vi "Ballard - 1553 Asynchronous RT Driver VI.vi"(10 "Parameters":variant, 11 "Process":refnum<class "Process.lvclass">) -> ()   [LabVIEW 2020, in "Ballard MIL-1553 Engine.lvlib"]
doc: "This VI is the Asynchronous VI for RT part."
uses:
  Ballard MIL-1553 Engine.lvlib
  <vilib>/NI/NIVS Inline Async API/_VS Inline Async API/Process/Process.lvclass
  <vilib>/NI/NIVS Inline Async API/_VS Inline Async API/Process/Process.lvclass/Process.ctl
  Controls/RT Async Data.ctl
  Controls/RT Async_Map BC2RT.ctl
  <vilib>/NI VeriStand/Custom Device API/Data Reference.ctl
  Controls/RT Async_Map_Type.ctl
  Controls/RT Async_Raw Values.ctl
  Controls/RT Async_Raw Values to Messages Index_Association.ctl
  Controls/Asynchronous - Parameter map_type.ctl
  Shared/EncodeDecode/_typedefs/parameter_config_type.ctl
  Shared/EncodeDecode/_typedefs/parameter_config_type_type.ctl
  Shared/EncodeDecode/_typedefs/parameter_config_encoding_type.ctl
  Controls/RT Async_Map RT2BC.ctl
  Controls/RT Async_Map RTs Status.ctl
  Controls/RT Async_Map BC Command Channels.ctl
  <vilib>/NI VeriStand/Custom Device API/Custom Device Item Ref.ctl
  Controls/RT Async_Map BC Acyclic Messages Trigger.ctl
  Controls/RT Async_Map RT Command Channels.ctl
  <vilib>/NI/NIVS Inline Async API/_Data Access Engine/Access Type Classes/Read/Read.lvclass/Read.ctl
  <vilib>/NI/NIVS Inline Async API/_Data Access Engine/Access Type Classes/ReadWrite/ReadWrite.lvclass/ReadWrite.ctl
  <vilib>/NI/NIVS Inline Async API/_Data Access Engine/Access Type Classes/Write/Write.lvclass/Write.ctl
  <vilib>/NI/NIVS Inline Async API/_Data Access Engine/Data Access Engine/Methods/Read.Data.Detect.vi
  <vilib>/NI/NIVS Inline Async API/_Data Access Engine/Data Access Engine/Methods/ReadWrite.Data.Read.vi
  <vilib>/NI/NIVS Inline Async API/_Data Access Engine/Data Access Engine/Methods/ReadWrite.Data.Reset.vi
  <vilib>/NI/NIVS Inline Async API/_Data Access Engine/Data Access Engine/Methods/Write.Data.vi
  <vilib>/NI/NIVS Inline Async API/_Data Access Engine/Data Access Engine/Methods/Read.Data.vi
  <vilib>/NI/NIVS Inline Async API/_VS Inline Async API/Process/Data Member Access/Read Data Access.vi
  <vilib>/NI/NIVS Inline Async API/_VS Inline Async API/Error Handling Process/SubVIs/Error.ConvertArray.vi
  <vilib>/NI/NIVS Inline Async API/_Data Access Engine/Access Type Classes/Read/Read.ProcessData.Detect.vi
  <vilib>/NI/NIVS Inline Async API/_Data Access Engine/Access Type Classes/ReadWrite/ReadWrite.ProcessData.Read.vi
  <vilib>/NI/NIVS Inline Async API/_Data Access Engine/Access Type Classes/ReadWrite/ReadWrite.ProcessData.Reset.vi
  <vilib>/NI/NIVS Inline Async API/_Data Access Engine/Access Type Classes/Write/Write.ProcessData.vi
  <vilib>/NI/NIVS Inline Async API/_Data Access Engine/Access Type Classes/Read/Read.ProcessData.vi
  <vilib>/NI/NIVS Inline Async API/_Data Access Engine/Access Type Classes/Write/Write.Buffer.vi
  <vilib>/NI/NIVS Inline Async API/_Data Access Engine/Access Type Classes/Write/Write.Commit.vi
  <vilib>/NI/NIVS Inline Async API/_Data Access Engine/Data Access Engine/Methods/Read.Lookup.vi
  <vilib>/NI/NIVS Inline Async API/_Data Access Engine/Data Access Engine/Methods/ReadWrite.Lookup.vi
  <vilib>/NI/NIVS Inline Async API/_Data Access Engine/Data Access Engine/Methods/Write.Lookup.vi
  <vilib>/NI/NIVS Inline Async API/_Data Access Engine/Data Access Engine/Data Access Engine.lvclass
  <vilib>/NI VeriStand/Custom Device API/Custom Device API.lvlib
panel:
  # "Custom Device Template\nv1.0"
  # "Use this template as a starting point for creating a custom device code module. The input controls shown here are specially named controls that the system will use to provide the device loop with data. The controls are not required for the device loop to run. For instance, if the device doesn't produce any output data, then you don't need the Device Outputs FIFO control. If you do use these controls, however, they need to have these exact names to be functional."
  # "The optional status notifier element is used to notify the RT engine of the last state of the custom device, and to indicate the device has completed execution. If this control is not used, a default No Error value is returned to the system when the device finishes execution.\n\nNote: This error state is not checked until the system shuts down. Use an output status channel to send more immediate status values to the system."
  # "This optional input can be used to send the VeriStand Engine the final status of the custom device initalization process. If this control exists on the custom device front panel, the VeriStand Engine will wait for a status update before starting up. If the custom device reports an error, that will abort the execution of the current configuration in the VeriStand Engine.\n\nThis control can be deleted if the custom device does not need to send the initialization status update."
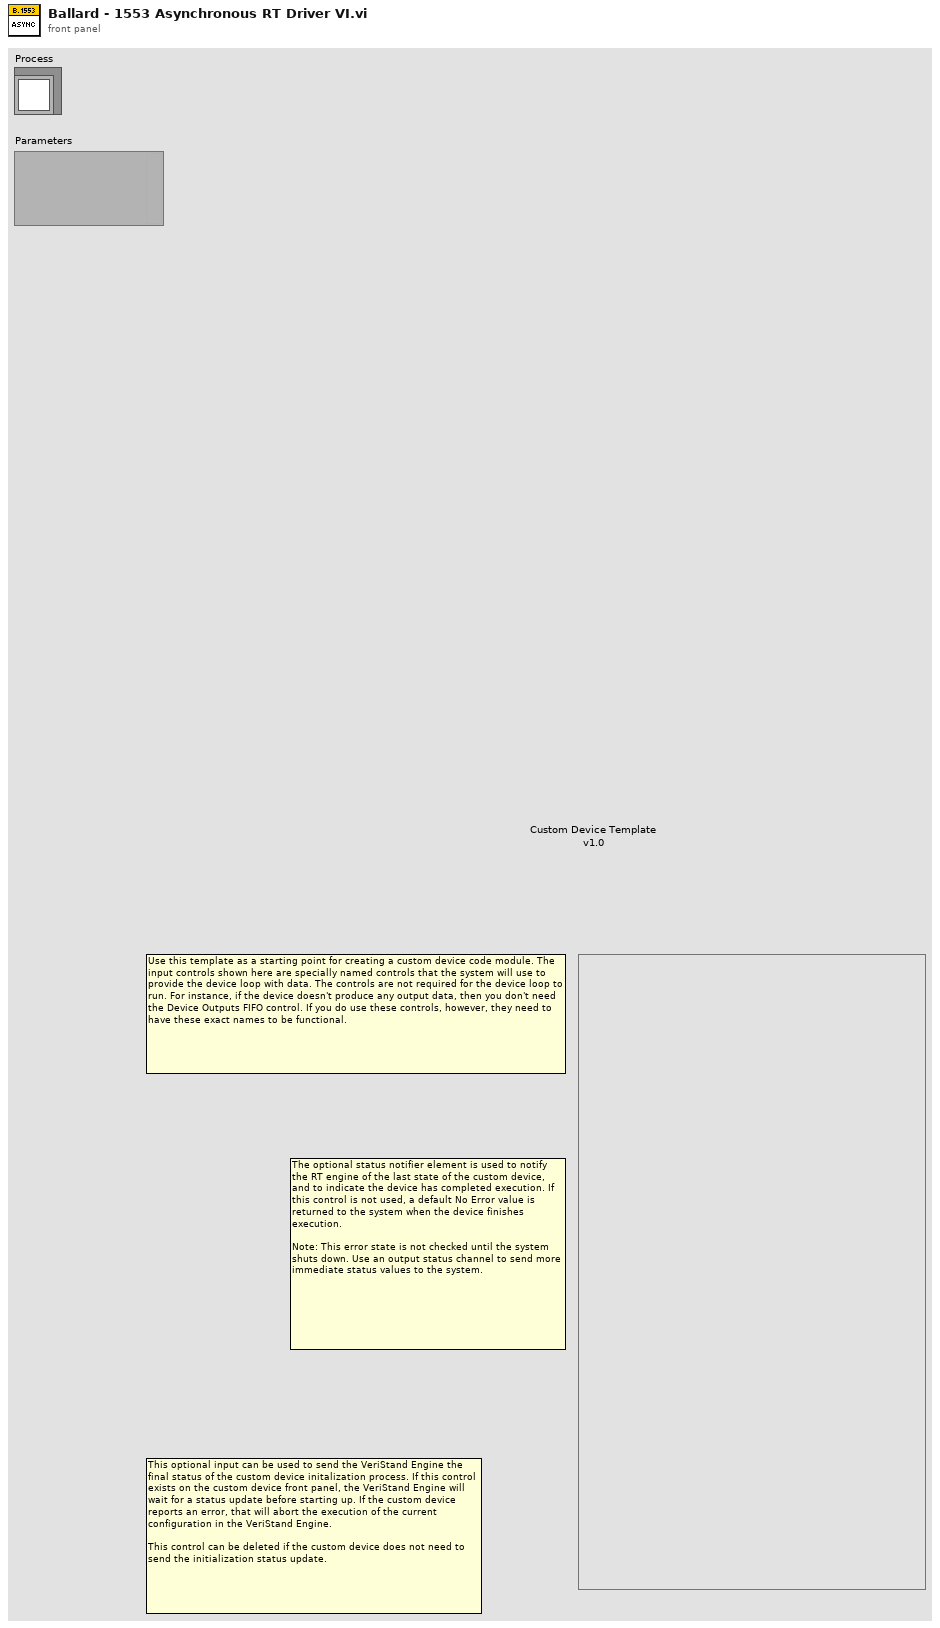
[diagram p1: front panel]
types:
  T1 = typedef "Ballard MIL-1553 Engine.lvlib/RT Async Data.ctl" = cluster{"Map (BC to RT)":T2[], "Raw Values (BC to RT)":T5, "param map (BC to RT)":T7, "Map (RT to ..)":T11[], "Raw Values (RT to ..)":T5, "param map (RT to BC)":T7, "Map (RTs Status)":T12[], "Raw Values (RTs Status)":T5, "Map (Bc Command Channels)":T13[], "MAP (BC Acyclic Messages Trigger)":T15[], "Map (RT Command Channels)":T16[], "Map (MC Rx)":T2[], "Raw Values (MC Rx)":T5, "param map (MC Rx)":T7, "Raw Values (MC Tx)":T5, "Map (MC Tx)":T11[], "param map (MC Tx)":T7}
  T2 = typedef "Ballard MIL-1553 Engine.lvlib/RT Async_Map BC2RT.ctl" = cluster{"Channel Index":i32, "ID":i32, "Channel Data Reference":T3, "Word Index":i32, "Message Handle":u64, "Type":T4, "Word Count":i32, "First Element Index":i32}
  T3 = typedef "Custom Device API.lvlib/Data Reference.ctl" = i32
  T4 = typedef "Ballard MIL-1553 Engine.lvlib/RT Async_Map_Type.ctl" = enum16{"Word (BC to RT)", "Word (MC (Rx))", "Acyclic Message Trigger", "Word (RT to ..)", "Word (RT to RT)", "Word (MC (Tx))", "RT Status", "BC Commands", "RT Commands"}
  T5 = typedef "Ballard MIL-1553 Engine.lvlib/RT Async_Raw Values.ctl" = cluster{"Association":T6[], "Raw Values Array":u16[]}
  T6 = typedef "Ballard MIL-1553 Engine.lvlib/RT Async_Raw Values to Messages Index_Association.ctl" = cluster{"Message Index":i32, "Raw Value Index":i32}
  T7 = typedef "Ballard MIL-1553 Engine.lvlib/Asynchronous - Parameter map_type.ctl" = cluster{"ParamConfig":T8[], "word_count":u8[]}
  T8 = typedef "parameter_config_type.ctl" = cluster{"Name":string, "Type":T9, "Units":string, "Nword":i32, "StartBit":i32, "Size":i32, "LSB_Value":i32, "Offset":i32, "Encoding":T10}
  T9 = typedef "parameter_config_type_type.ctl" = enum16{"Opaque", "Enum", "Float", "Integer", "Bcd", "Bool"}
  T10 = typedef "parameter_config_encoding_type.ctl" = enum16{"None", "2-complement", "Unsigned"}
  T11 = typedef "Ballard MIL-1553 Engine.lvlib/RT Async_Map RT2BC.ctl" = cluster{"Channel Index":i32, "ID":i32, "Word Data Reference":T3, "First element Index":i32, "rt Transfer Handle":u64, "Type":T4, "Word Count":i32}
  T12 = typedef "Ballard MIL-1553 Engine.lvlib/RT Async_Map RTs Status.ctl" = cluster{"Channel Index":i32, "ID":i32, "rt Transfer Handle":u64, "Type":T4}
  T13 = typedef "Ballard MIL-1553 Engine.lvlib/RT Async_Map BC Command Channels.ctl" = cluster{"Channel Index":i32, "ID":i32, "BC Handle":u64, "Type":T4, "BC Command Channel Ref":T14, "Command Type":enum16{"Start Command", "Stop Command"}}
  T14 = typedef "Custom Device API.lvlib/Custom Device Item Ref.ctl" = u64
  T15 = typedef "Ballard MIL-1553 Engine.lvlib/RT Async_Map BC Acyclic Messages Trigger.ctl" = cluster{"Channel Index":i32, "BC Handle":u64, "Type":T4, "Acyclic Message Trigger Channel Ref":T14, "Message Name":string}
  T16 = typedef "Ballard MIL-1553 Engine.lvlib/RT Async_Map RT Command Channels.ctl" = cluster{"Channel Index":i32, "ID":i32, "RT Handle":u64, "Type":T4, "RT Command Channel Ref":T14, "Command Type":enum16{"Start Command", "Stop Command"}}
  T17 = typedef "Data Access Engine.lvlib/Data Access Engine.lvclass/Read.DVR.ctl" = refnum<data-value>
  T18 = typedef "Data Access Engine.lvlib/Data Access Engine.lvclass/ReadWrite.DVR.ctl" = refnum<data-value>
  T19 = typedef "Data Access Engine.lvlib/Data Access Engine.lvclass/Write.DVR.ctl" = refnum<data-value>
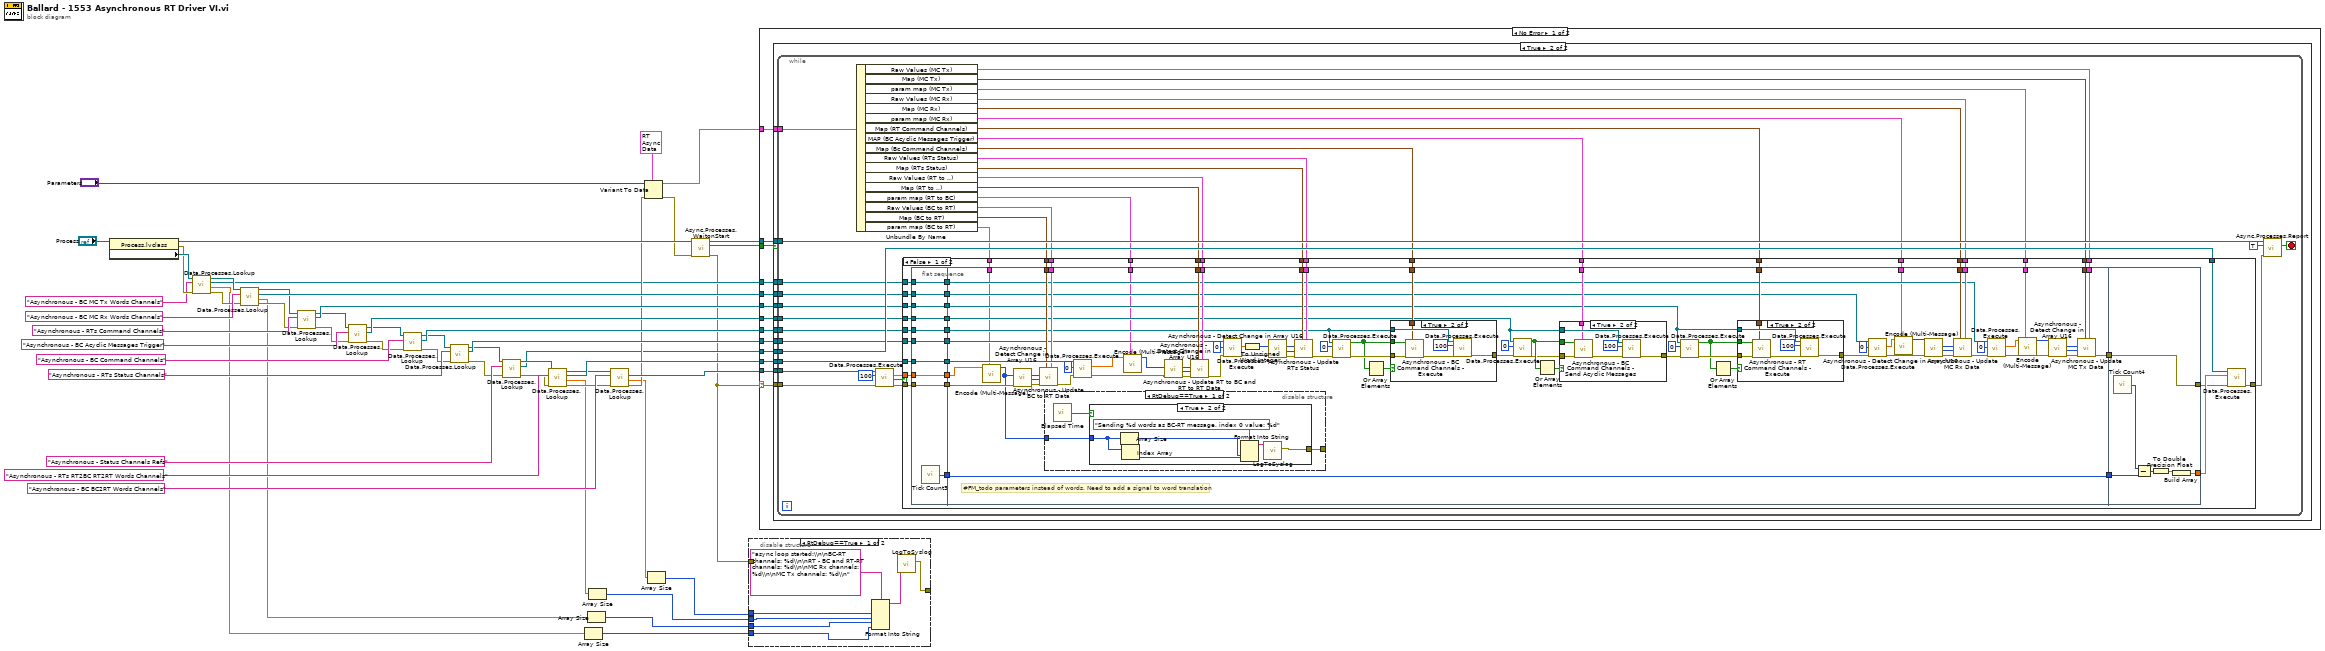
[diagram p0: block diagram]
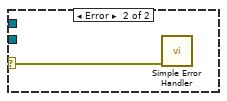
[diagram p10: hidden frame]
diagram:
  n1 = property class="Process.lvclass"(reference="Process") -> (reference out=w50:refnum<class "Process.lvclass">, error out=w15:errorcluster, "Data Member Access:Data Access"=w16:refnum<class "Data Access Engine.lvclass">)  [unwired: 1 in]
  n2 = call-poly <vilib>:"Data.Processes.Lookup.vi"("error in (no error)"=w15, "Name"="Asynchronous - BC MC Tx Words Channels", "Data Access API in"=w16) -> ("error out"=w14:errorcluster, "Initial Values"=w8:dbl[], "Ref"=w12:T17, "Data Access API out"=w13:refnum<class "Data Access Engine.lvclass">)  [unwired: 5 in]
  n3 = call-poly <vilib>:"Data.Processes.Lookup.vi"("error in (no error)"=w14, "Name"="Asynchronous - BC MC Rx Words Channels", "Data Access API in"=w13) -> ("error out"=w17:errorcluster, "Initial Values"=w7:dbl[], "Ref"=w32:T17, "Data Access API out"=w18:refnum<class "Data Access Engine.lvclass">)  [unwired: 5 in]
  n4 = call-poly <vilib>:"Data.Processes.Lookup.vi"("error in (no error)"=w17, "Name"="Asynchronous - RTs Command Channels", "Data Access API in"=w18) -> ("error out"=w19:errorcluster, "Ref"=w34:T18, "Data Access API out"=w20:refnum<class "Data Access Engine.lvclass">)  [unwired: 5 in, 1 out]
  n5 = call-poly <vilib>:"Data.Processes.Lookup.vi"("error in (no error)"=w19, "Name"="Asynchronous - BC Acyclic Messages Trigger", "Data Access API in"=w20) -> ("error out"=w22:errorcluster, "Ref"=w36:T18, "Data Access API out"=w21:refnum<class "Data Access Engine.lvclass">)  [unwired: 5 in, 1 out]
  n6 = call-poly <vilib>:"Data.Processes.Lookup.vi"("error in (no error)"=w22, "Name"="Asynchronous - BC Command Channels", "Data Access API in"=w21) -> ("error out"=w23:errorcluster, "Ref"=w38:T18, "Data Access API out"=w24:refnum<class "Data Access Engine.lvclass">)  [unwired: 5 in, 1 out]
  n7 = call-poly <vilib>:"Data.Processes.Lookup.vi"("error in (no error)"=w23, "Name"="Asynchronous - RTs Status Channels", "Data Access API in"=w24) -> ("error out"=w25:errorcluster, "Ref"=w40:T17, "Data Access API out"=w26:refnum<class "Data Access Engine.lvclass">)  [unwired: 5 in, 1 out]
  n8 = call-poly <vilib>:"Data.Processes.Lookup.vi"("error in (no error)"=w25, "Name"="Asynchronous - Status Channels Refs", "Data Access API in"=w26) -> ("error out"=w27:errorcluster, "Ref"=w10:T19, "Data Access API out"=w28:refnum<class "Data Access Engine.lvclass">)  [unwired: 5 in, 1 out]
  n9 = call-poly <vilib>:"Data.Processes.Lookup.vi"("error in (no error)"=w27, "Name"="Asynchronous - RTs RT2BC RT2RT Words Channels", "Data Access API in"=w28) -> ("error out"=w29:errorcluster, "Initial Values"=w6:dbl[], "Ref"=w46:T17, "Data Access API out"=w44:refnum<class "Data Access Engine.lvclass">)  [unwired: 5 in]
  n10 = Array Size(array=w8) -> (size(s)=w1:i32)
  n11 = Array Size(array=w7) -> (size(s)=w2:i32)
  n12 = Array Size(array=w6) -> (size(s)=w3:i32)
  n13 = call-poly <vilib>:"Data.Processes.Lookup.vi"("error in (no error)"=w29, "Name"="Asynchronous - BC BC2RT Words Channels", "Data Access API in"=w44) -> ("error out"=w30:errorcluster, "Initial Values"=w5:dbl[], "Ref"=w52:T17)  [unwired: 5 in, 1 out]
  n14 = Variant To Data(error in=w30, type=T1 {"Map (BC to RT)"=[], "Raw Values (BC to RT)"={"Association"=[], "Raw Values Array"=[]}, "param map (BC to RT)"={"ParamConfig"=[], "word_count"=[]}, "Map (RT to ..)"=[], "Raw Values (RT to ..)"={"Association"=[], "Raw Values Array"=[]}, "param map (RT to BC)"={"ParamConfig"=[], "word_count"=[]}, "Map (RTs Status)"=[], "Raw Values (RTs Status)"={"Association"=[], "Raw Values Array"=[]}, "Map (Bc Command Channels)"=[], "MAP (BC Acyclic Messages Trigger)"=[], "Map (RT Command Channels)"=[], "Map (MC Rx)"=[], "Raw Values (MC Rx)"={"Association"=[], "Raw Values Array"=[]}, "param map (MC Rx)"={"ParamConfig"=[], "word_count"=[]}, "Raw Values (MC Tx)"={"Association"=[], "Raw Values Array"=[]}, "Map (MC Tx)"=[], "param map (MC Tx)"={"ParamConfig"=[], "word_count"=[]}} ("RT Async Data"), Variant="Parameters") -> (data=w45:T1, error out=w31:errorcluster)
  n15 = Array Size(array=w5) -> (size(s)=w4:i32)
  n16 = call <vilib>:"Async.Processes.WaitonStart.vi"("error in (no error)"=w31, "Process"=w50) -> ("error out"=w9:errorcluster, "Execute"=w54:bool, "Process out"=w53:refnum<class "Process.lvclass">)  [unwired: 7 in]
  n17 = disable-structure shown="RtDebug==True" {
    disable-tunnel: [w59 _] -> _
    disable-tunnel: w9 -> [_ _]
    disable-tunnel: w4 -> [w58 _]
    disable-tunnel: w3 -> [w57 _]
    disable-tunnel: w2 -> [w56 _]
    disable-tunnel: w1 -> [w55 _]
    frame condition #0 (active) {
      n18 = Format Into String(format string="async loop started:\\n\nBC-RT channels: %d\\n\nRT - BC and RT-RT channels: %d\\n\nMC Rx channels: %d\\n\nMC Tx channels: %d\\n", w58, w57, w56, w55) -> (resulting string=w61:string)  [unwired: 2 in, 1 out]
      n19 = call "LogToSyslog.vi"("message"=w61) -> ("error out"=w59:errorcluster)  [unwired: 9 in, 1 out]
    }
    frame condition #1 {
    }
  }
  n20 = case shown="No Error" w9 {
    selector: w9 -> [w70 w294]
    tunnel: w54 -> [w74 _]
    tunnel: w53 -> [w73 _]
    tunnel: w10 -> [w72 _]
    tunnel: w52 -> [w71 _]
    tunnel: w45 -> [w69 _]
    tunnel: w46 -> [w68 _]
    tunnel: w40 -> [w67 _]
    tunnel: w38 -> [w66 _]
    tunnel: w36 -> [w65 _]
    tunnel: w34 -> [w64 _]
    tunnel: w32 -> [w63 _]
    tunnel: w12 -> [w62 _]
    frame No Error {
      n21 = case shown="True" w74 {
        tunnel: w70 -> [_ w83]
        tunnel: w73 -> [_ w84]
        tunnel: w71 -> [_ w86]
        tunnel: w72 -> [_ w85]
        tunnel: w69 -> [_ w82]
        tunnel: w68 -> [_ w81]
        tunnel: w67 -> [_ w80]
        tunnel: w66 -> [_ w79]
        tunnel: w65 -> [_ w78]
        tunnel: w64 -> [_ w77]
        tunnel: w63 -> [_ w76]
        tunnel: w62 -> [_ w75]
        frame False {
        }
        frame True {
          n22 = while {
            tunnel: w83 -> [w118]
            tunnel: w84 -> [w122]
            tunnel: w86 -> [w120]
            tunnel: w85 -> [w119]
            tunnel: w82 -> [w115]
            tunnel: w81 -> [w114]
            tunnel: w80 -> [w107]
            tunnel: w79 -> [w104]
            tunnel: w78 -> [w102]
            tunnel: w77 -> [w100]
            tunnel: w76 -> [w98]
            tunnel: w75 -> [w93]
            stop <- w121 stop-if-true
            n23 = Unbundle By Name(w115) -> ("Raw Values (MC Tx)"=w91:T5, "Map (MC Tx)"=w92:T11[], "param map (MC Tx)"=w87:T7, "Raw Values (MC Rx)"=w95:T5, "Map (MC Rx)"=w94:T2[], "param map (MC Rx)"=w88:T7, "Map (RT Command Channels)"=w99:T16[], "MAP (BC Acyclic Messages Trigger)"=w101:T15[], "Map (Bc Command Channels)"=w103:T13[], "Raw Values (RTs Status)"=w105:T5, "Map (RTs Status)"=w106:T12[], "Raw Values (RT to ..)"=w110:T5, "Map (RT to ..)"=w111:T11[], "param map (RT to BC)"=w89:T7, "Raw Values (BC to RT)"=w108:T5, "Map (BC to RT)"=w109:T2[], "param map (BC to RT)"=w90:T7)
            n24 = call-poly <vilib>:"Data.Processes.Execute.vi"("error in (no error)"=w118, "timeout ms"=100, "Ref"=w120) -> ("error out"=w116:errorcluster, "Timeout?"=w113:bool, "Values"=w117:dbl[])  [unwired: 6 in]
            n25 = case shown="False" w113 {
              tunnel: w119 -> [w159 _]
              tunnel: [w158 w293] -> w97
              tunnel: w117 -> [w157 _]
              tunnel: w116 -> [w156 w293]
              tunnel: w114 -> [w154 _]
              tunnel: w111 -> [w153 _]
              tunnel: w110 -> [w152 _]
              tunnel: w109 -> [w151 _]
              tunnel: w108 -> [w150 _]
              tunnel: w107 -> [w149 _]
              tunnel: w106 -> [w147 _]
              tunnel: w105 -> [w146 _]
              tunnel: w104 -> [w145 _]
              tunnel: w103 -> [w142 _]
              tunnel: w102 -> [w141 _]
              tunnel: w101 -> [w139 _]
              tunnel: w100 -> [w138 _]
              tunnel: w99 -> [w136 _]
              tunnel: w98 -> [w135 _]
              tunnel: w95 -> [w132 _]
              tunnel: w94 -> [w131 _]
              tunnel: w93 -> [w130 _]
              tunnel: w92 -> [w128 _]
              tunnel: w91 -> [w127 _]
              tunnel: w90 -> [w126 _]
              tunnel: w89 -> [w125 _]
              tunnel: w88 -> [w124 _]
              tunnel: w87 -> [w123 _]
              frame False {
                n26 = flat-sequence {
                  tunnel: w157 -> [w173]
                  tunnel: w156 -> [w174]
                  tunnel: [w174] -> w164
                  tunnel: [w173] -> w163
                  tunnel: [w172] -> w162
                  tunnel: w154 -> [w171]
                  tunnel: [w171] -> w161
                  tunnel: w149 -> [w170]
                  tunnel: [w170] -> w148
                  tunnel: w145 -> [w169]
                  tunnel: [w169] -> w144
                  tunnel: w141 -> [w168]
                  tunnel: [w168] -> w140
                  tunnel: w138 -> [w167]
                  tunnel: [w167] -> w137
                  tunnel: w135 -> [w166]
                  tunnel: [w166] -> w134
                  tunnel: w130 -> [w165]
                  tunnel: [w165] -> w129
                  tunnel: w164 -> [w249]
                  tunnel: w163 -> [w184]
                  tunnel: w162 -> [w253]
                  tunnel: [w253] -> w160
                  tunnel: w161 -> [w252]
                  tunnel: w153 -> [w251]
                  tunnel: w152 -> [w250]
                  tunnel: w151 -> [w245]
                  tunnel: w150 -> [w244]
                  tunnel: w148 -> [w242]
                  tunnel: w147 -> [w241]
                  tunnel: w146 -> [w240]
                  tunnel: w144 -> [w239]
                  tunnel: w142 -> [w238]
                  tunnel: w140 -> [w237]
                  tunnel: w139 -> [w236]
                  tunnel: w137 -> [w235]
                  tunnel: w136 -> [w234]
                  tunnel: w134 -> [w233]
                  tunnel: [w188] -> w133
                  tunnel: w132 -> [w197]
                  tunnel: w131 -> [w196]
                  tunnel: w129 -> [w187]
                  tunnel: w128 -> [w186]
                  tunnel: w127 -> [w185]
                  tunnel: w126 -> [w183]
                  tunnel: w125 -> [w180]
                  tunnel: w124 -> [w178]
                  tunnel: w123 -> [w176]
                  tunnel: w160 -> [w292]
                  tunnel: [w288] -> w155
                  tunnel: [w287] -> w143
                  tunnel: w133 -> [w287]
                  frame #0 {
                    n27 = call "Tick Count3"() -> ("Tick Count(uSec)"=w172:u32)
                  }
                  frame #1 {
                    # "#FM_todo parameters instead of words. Need to add a signal to word translation"
                    n28 = call "Encode (Multi-Message).vi"("param map"=w183, "parameters in"=w184) -> ("words out"=w175:u16[])  [unwired: 9 in]
                    n29 = call "Asynchronous - Detect Change in Array U16.vi"("Error (in)"=w249, "Data (in)"=w175) -> ("Error (out)"=w248:errorcluster, "Indexes"=w246:i32[], "Data (out)"=w247:u16[])  [unwired: 7 in]
                    n30 = call "Asynchronous - Update BC to RT Data.vi"("Raw Values (BC to RT)"=w244, "Map (BC to RT)"=w245, "Error (in)"=w248, "Updated FIFO Index []"=w246, "U16 []"=w247) -> ("Error (out)"=w243:errorcluster)  [unwired: 6 in]
                    n31 = disable-structure shown="RtDebug==True" {
                      disable-tunnel: [w256 _] -> _
                      disable-tunnel: w175 -> [w254 _]
                      frame condition #0 (active) {
                        n32 = call "Elapsed Time"() -> ("Time has Elapsed"=w255:bool)  [unwired: 12 in, 7 out]
                        n33 = case shown="True" w255 {
                          tunnel: [_ w260] -> w256
                          tunnel: w254 -> [_ w259]
                          frame False {
                          }
                          frame True {
                            n34 = Array Size(array=w259) -> (size(s)=w257:i32)
                            n35 = Index Array(array=w259) -> (element=w258:u16)  [unwired: 1 in]
                            n36 = Format Into String(format string="Sending %d words as BC-RT message. index 0 value: %d", w257, w258) -> (resulting string=w262:string)  [unwired: 2 in, 1 out]
                            n37 = call "LogToSyslog.vi"("message"=w262) -> ("error out"=w260:errorcluster)  [unwired: 9 in, 1 out]
                          }
                        }
                      }
                      frame condition #1 {
                      }
                    }
                    n38 = call-poly <vilib>:"Data.Processes.Execute.vi"("error in (no error)"=w243, "timeout ms"=0, "Ref"=w252) -> ("error out"=w231:errorcluster, "Values"=w182:dbl[])  [unwired: 5 in, 2 out]
                    n39 = call "Encode (Multi-Message).vi"("param map"=w180, "parameters in"=w182) -> ("words out"=w181:u16[])  [unwired: 9 in]
                    n40 = call "Asynchronous - Detect Change in Array U16.vi"("Error (in)"=w231, "Data (in)"=w181) -> ("Error (out)"=w230:errorcluster, "Indexes"=w229:i32[], "Data (out)"=w228:u16[])  [unwired: 7 in]
                    n41 = call "Asynchronous - Update RT to BC and RT to RT Data.vi"("Raw Values (RT to BC)"=w250, "Map (RT to BC)"=w251, "Error (in)"=w230, "Updated FIFO Index []"=w229, "U16 []"=w228) -> ("Error (out)"=w227:errorcluster)  [unwired: 6 in]
                    n42 = call-poly <vilib>:"Data.Processes.Execute.vi"("error in (no error)"=w227, "timeout ms"=0, "Ref"=w242) -> ("error out"=w223:errorcluster, "Values"=w225:dbl[])  [unwired: 5 in, 2 out]
                    n43 = To Unsigned Word Integer(number=w225) -> (unsigned 16bit integer=w224:u16[])
                    n44 = call "Asynchronous - Detect Change in Array U16.vi"("Error (in)"=w223, "Data (in)"=w224) -> ("Error (out)"=w222:errorcluster, "Indexes"=w220:i32[], "Data (out)"=w221:u16[])  [unwired: 7 in]
                    n45 = call "Asynchronous - Update RTs Status.vi"("Raw Values (RTs Status)"=w240, "Map (RTs Status)"=w241, "Error (in)"=w222, "Updated FIFO Index []"=w220, "U16 []"=w221) -> ("Error (out)"=w218:errorcluster)  [unwired: 6 in]
                    n46 = call-poly <vilib>:"Data.Processes.Execute.vi"("error in (no error)"=w218, "timeout ms"=0, "Ref"=w239) -> ("error out"=w216:errorcluster, "Detect?"=w215:bool[])  [unwired: 5 in, 2 out]
                    n47 = Or Array Elements(Boolean array=w215) -> (logical OR=w217:bool)
                    n48 = case shown="True" w217 {
                      tunnel: w216 -> [w279 w283]
                      tunnel: w239 -> [_ w285]
                      tunnel: w215 -> [_ w281]
                      tunnel: [w279 w284] -> w214
                      tunnel: w238 -> [_ w280]
                      frame False {
                      }
                      frame True {
                        n49 = call "Asynchronous - BC Command Channels - Execute.vi"("Map (Bc Command Channels)"=w280, "Error (in)"=w283, "Changes?"=w281) -> ("Error (out)"=w282:errorcluster)  [unwired: 8 in]
                        n50 = call-poly <vilib>:"Data.Processes.Execute.vi"("error in (no error)"=w282, "timeout ms"=100, "Ref"=w285) -> ("error out"=w284:errorcluster)  [unwired: 7 in, 1 out]
                      }
                    }
                    n51 = call-poly <vilib>:"Data.Processes.Execute.vi"("error in (no error)"=w214, "timeout ms"=0, "Ref"=w237) -> ("error out"=w211:errorcluster, "Detect?"=w212:bool[])  [unwired: 5 in, 2 out]
                    n52 = Or Array Elements(Boolean array=w212) -> (logical OR=w210:bool)
                    n53 = case shown="True" w210 {
                      tunnel: w211 -> [w271 w275]
                      tunnel: w237 -> [_ w277]
                      tunnel: w212 -> [_ w273]
                      tunnel: [w271 w276] -> w206
                      tunnel: w236 -> [_ w272]
                      frame False {
                      }
                      frame True {
                        n54 = call "Asynchronous - BC Command Channels - Send Acyclic Messages.vi"("Map (Bc Acyclic Messages Trigger)"=w272, "Error (in)"=w275, "Changes?"=w273) -> ("Error (out)"=w274:errorcluster)  [unwired: 8 in]
                        n55 = call-poly <vilib>:"Data.Processes.Execute.vi"("error in (no error)"=w274, "timeout ms"=100, "Ref"=w277) -> ("error out"=w276:errorcluster)  [unwired: 7 in, 1 out]
                      }
                    }
                    n56 = call-poly <vilib>:"Data.Processes.Execute.vi"("error in (no error)"=w206, "timeout ms"=0, "Ref"=w235) -> ("error out"=w208:errorcluster, "Detect?"=w207:bool[])  [unwired: 5 in, 2 out]
                    n57 = Or Array Elements(Boolean array=w207) -> (logical OR=w205:bool)
                    n58 = case shown="True" w205 {
                      tunnel: w208 -> [w263 w267]
                      tunnel: w235 -> [_ w269]
                      tunnel: w207 -> [_ w265]
                      tunnel: [w263 w268] -> w204
                      tunnel: w234 -> [_ w264]
                      frame False {
                      }
                      frame True {
                        n59 = call "Asynchronous - RT Command Channels - Execute.vi"("Map (RT Command Channels)"=w264, "Error (in)"=w267, "Changes?"=w265) -> ("Error (out)"=w266:errorcluster)  [unwired: 8 in]
                        n60 = call-poly <vilib>:"Data.Processes.Execute.vi"("error in (no error)"=w266, "timeout ms"=100, "Ref"=w269) -> ("error out"=w268:errorcluster)  [unwired: 7 in, 1 out]
                      }
                    }
                    n61 = call-poly <vilib>:"Data.Processes.Execute.vi"("error in (no error)"=w204, "timeout ms"=0, "Ref"=w233) -> ("error out"=w202:errorcluster, "Values"=w179:dbl[])  [unwired: 5 in, 2 out]
                    n62 = call "Encode (Multi-Message).vi"("param map"=w178, "parameters in"=w179) -> ("words out"=w201:u16[])  [unwired: 9 in]
                    n63 = call "Asynchronous - Detect Change in Array U16.vi"("Error (in)"=w202, "Data (in)"=w201) -> ("Error (out)"=w200:errorcluster, "Indexes"=w199:i32[], "Data (out)"=w198:u16[])  [unwired: 7 in]
                    n64 = call "Asynchronous - Update MC Rx Data.vi"("Raw Values (MC Rx)"=w197, "Map (MC Rx)"=w196, "Error (in)"=w200, "Updated FIFO Index []"=w199, "U16 []"=w198) -> ("Error (out)"=w189:errorcluster)  [unwired: 6 in]
                    n65 = call-poly <vilib>:"Data.Processes.Execute.vi"("error in (no error)"=w189, "timeout ms"=0, "Ref"=w187) -> ("error out"=w191:errorcluster, "Values"=w177:dbl[])  [unwired: 5 in, 2 out]
                    n66 = call "Encode (Multi-Message).vi"("param map"=w176, "parameters in"=w177) -> ("words out"=w192:u16[])  [unwired: 9 in]
                    n67 = call "Asynchronous - Detect Change in Array U16.vi"("Error (in)"=w191, "Data (in)"=w192) -> ("Error (out)"=w193:errorcluster, "Indexes"=w194:i32[], "Data (out)"=w195:u16[])  [unwired: 7 in]
                    n68 = call "Asynchronous - Update MC Tx Data.vi"("Raw Values (MC Tx)"=w185, "Map (MC Tx)"=w186, "Error (in)"=w193, "Updated FIFO Index []"=w194, "U16 []"=w195) -> ("Error (out)"=w188:errorcluster)  [unwired: 6 in]
                  }
                  frame #2 {
                    n69 = call "Tick Count4"() -> ("Tick Count(uSec)"=w291:u32)
                    n70 = Subtract(x=w291, y=w292) -> (x-y=w290:u32)
                    n71 = To Double Precision Float(number=w290) -> (double precision float=w289:dbl)
                    n72 = Build Array(w289) -> (w288:dbl[])
                  }
                }
                n73 = call-poly <vilib>:"Data.Processes.Execute.vi"("error in (no error)"=w143, "Values"=w155, "Ref"=w159) -> ("error out"=w158:errorcluster)  [unwired: 8 in]
              }
              frame True {
              }
            }
            n74 = call <vilib>:"Async.Processes.Report.vi"("Error"=w97, "Stop Async on Error?"=TRUE, "Process in"=w122) -> ("Stop"=w121:bool)  [unwired: 7 in, 1 out]
          }
        }
      }
    }
    frame Error {
      n75 = call <vilib>:"Simple Error Handler.vi"("error in (no error)"=w294) -> ()  [unwired: 4 in, 5 out]
    }
  }
